vi "NetTTLSend.vi"(8 "error in":errorcluster, 9 "channel":u16=1, 10 "turn on?":bool=TRUE, 11 "socket in":refnum<class "zmq_socket.lvclass">) -> (0 "error out":errorcluster, 3 "socket out":refnum<class "zmq_socket.lvclass">)   [LabVIEW 2017]
uses:
  <vilib>/addons/zeromq/zmq_socket.lvclass
  <vilib>/Utility/error.llb/Error Cluster From Error Code.vi
  <vilib>/ErrorRing/Error Ring.xnode
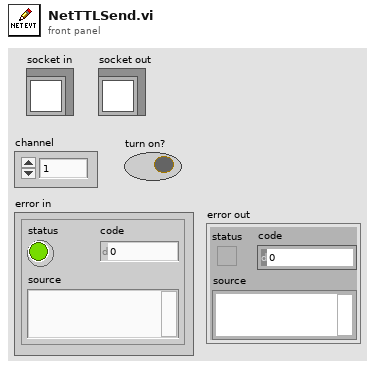
[diagram p1: front panel]
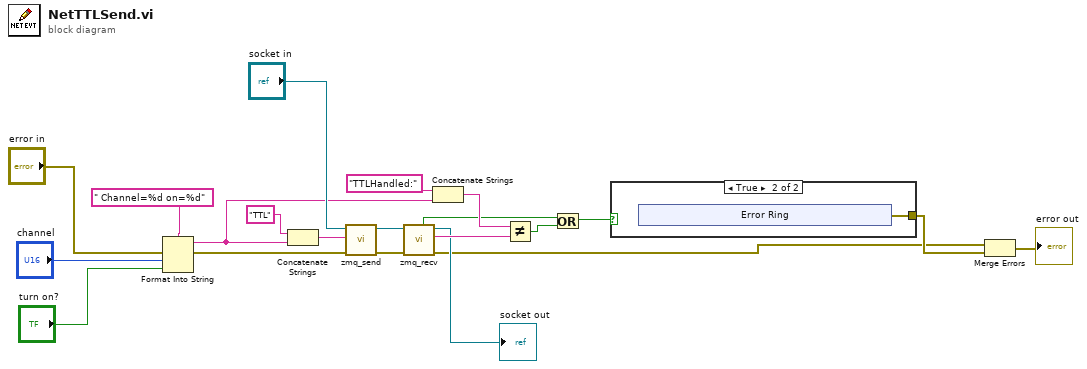
[diagram p0: block diagram]
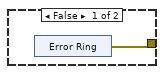
[diagram p2: hidden frame]
diagram:
  n1 = Format Into String(format string=" Channel=%d on=%d" ("initial string"), error in="error in", "channel", "turn on?") -> (resulting string=w10:string, error out=w17:errorcluster)  [unwired: 1 in]
  n2 = Concatenate Strings("TTL" ("string"), w10) -> (w14:string)
  n3 = call <vilib>:"zmq_send.vi"("error in"=w17, "data"=w14, "socket in"="socket in") -> ("error out"=w13:errorcluster, "socket out"=w12:refnum<class "zmq_socket.lvclass">)  [unwired: 4 in]
  n4 = call <vilib>:"zmq_recv.vi"("error in"=w13, "socket in"=w12) -> ("error out"=w1:errorcluster, "data"=w8:string, "socket out"=→"socket out":refnum<class "zmq_socket.lvclass">, "timeout?"=w6:bool)  [unwired: 3 in, 1 out]
  n5 = Concatenate Strings("TTLHandled:" ("string"), w10) -> (w11:string)
  n6 = Not Equal?(x=w11, y=w8) -> (x != y?=w5:bool)
  n7 = Or(x=w6, y=w5) -> (x .or. y?=w4:bool)
  n8 = case shown="True" w4 {
    tunnel: [w22 w24] -> w2
    frame False {
      n9 = xnode "Error Ring"() -> ("error out"=w22:errorcluster)
    }
    frame True {
      n10 = xnode "Error Ring"() -> ("error out"=w24:errorcluster)
    }
  }
  n11 = Merge Errors(w1, w2) -> (→"error out":errorcluster)
